vi "GetUser.vi"(10 "string":string caption="字符串", 11 "权限":string(combo)="QX01") -> (0 "员工姓名":string, 1 "权限":bool, 3 "员工ID":string)   [LabVIEW 2013]
uses:
  <vilib>/Utility/error.llb/whitespace.ctl
panel:
  in  "error in (no error)":errorcluster
  out "error out":errorcluster
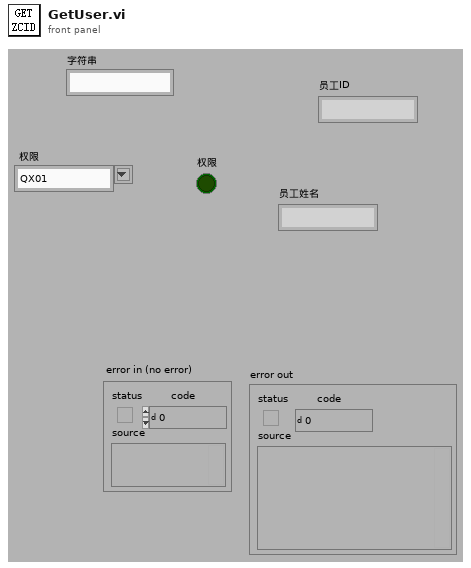
[diagram p1: front panel]
types:
  T1 = typedef "whitespace.ctl" = u16
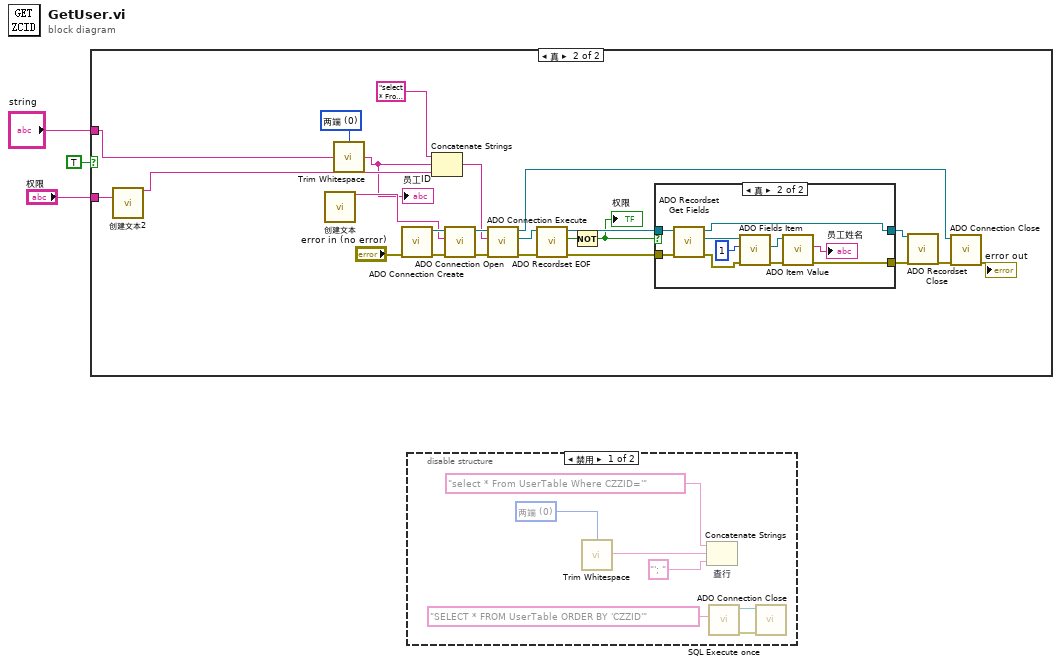
[diagram p0: block diagram]
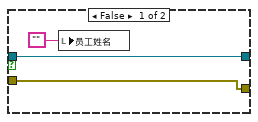
[diagram p3: hidden frame]
diagram:
  n1 = case shown="真" TRUE {
    tunnel: "权限" -> [_ w6]
    tunnel: "string" -> [_ w4]
    frame False {
    }
    frame True {
      w20 = T1 0 items=["两端", "字符串首端", "字符串末端"] ("location (both)")
      n2 = call "创建文本2"("权限"=w6) -> ("Result"=w7:string)  [unwired: 13 in, 1 out]
      n3 = call "创建文本"() -> ("Result"=w9:string)  [unwired: 14 in, 1 out]
      n4 = call <vilib>:"Trim Whitespace.vi"("string"=w4, "location (both)"=w20) -> ("trimmed string"=w5:string)
      "员工ID" <- w5
      n5 = call "ADO Connection Create.vi"("error in (no error)"="error in (no error)") -> ("error out"=w26:errorcluster, "ADODB._Connection Out"=w27:refnum<k7>)  [unwired: 9 out]
      n6 = Concatenate Strings ("查位置")("select * From UserTable Where  CZZID='" ("字符串 2"), w5, w7) -> (w10:string)
      n7 = call "ADO Connection Open.vi"("error in (no error)"=w26, "ConnectionString"=w9, "ADODB._Connection In"=w27) -> ("error out"=w25:errorcluster, "ADODB._Connection Out"=w11:refnum<k7>)  [unwired: 7 out]
      n8 = call "ADO Connection Execute.vi"("error in (no error)"=w25, "CommandText"=w10, "ADODB._Connection In"=w11) -> ("error out"=w23:errorcluster, "RecordSet"=w24:refnum<k7>, "ADODB._Connection Out"=w12:refnum<k7>)  [unwired: 6 out]
      n9 = call "ADO Recordset EOF.vi"("error in (no error)"=w23, "ADODB._Recordset In"=w24) -> ("error out"=w16:errorcluster, "EOF"=w13:bool, "ADODB._Recordset Out"=w17:refnum<k7>)  [unwired: 7 out]
      n10 = Not(x=w13) -> (.not. x?=w8:bool)
      "权限" <- w8
      n11 = case shown="真" w8 {
        tunnel: w17 -> [w29 w40]
        tunnel: w16 -> [w30 w39]
        tunnel: [w29 w38] -> w15
        tunnel: [w30 w32] -> w14
        frame False {
          n12 = local write "员工姓名"("") -> ()
        }
        frame True {
          n13 = call "ADO Recordset Get Fields.vi"("error in (no error)"=w39, "ADODB._Recordset In"=w40) -> ("error out"=w31:errorcluster, "Fields Out"=w37:refnum<k7>, "ADODB._Recordset Out"=w38:refnum<k7>)  [unwired: 7 out]
          n14 = call "ADO Fields Item.vi"("error in (no error)"=w31, "Index"=1, "Fields In"=w37) -> ("error out"=w35:errorcluster, "Item Out"=w34:refnum<k7>)  [unwired: 7 out]
          n15 = call "ADO Item Value.vi"("error in (no error)"=w35, "Item In"=w34) -> ("error out"=w32:errorcluster, "Value"=→"员工姓名":string)  [unwired: 8 out]
        }
      }
      n16 = call "ADO Recordset Close.vi"("ADODB._Recordset In"=w15, "error in (no error)"=w14) -> ("error out"=w22:errorcluster)  [unwired: 17 out]
      n17 = call "ADO Connection Close.vi"("error in (no error)"=w22, "ADODB._Connection In"=w12) -> ("error out"=→"error out":errorcluster)  [unwired: 9 out]
    }
  }
  n18 = disable-structure shown="禁用" {
    frame Disabled {
      w44 = T1 0 items=["两端", "字符串首端", "字符串末端"] ("location (both)")
      n19 = call <vilib>:"Trim Whitespace.vi"("location (both)"=w44) -> ("trimmed string"=w43:string)  [unwired: 1 in]
      n20 = Concatenate Strings "查行"("select * From UserTable Where CZZID='" ("字符串 2"), w43, "'; " ("字符串 2")) -> ()  [unwired: 1 out]
      n21 = call "SQL Execute once.vi"("Command Text"="SELECT * FROM UserTable ORDER BY 'CZZID'") -> ("error out"=w47:errorcluster, "ADODB._Connection Out"=w46:refnum<k7>)  [unwired: 3 in, 6 out]
      n22 = call "ADO Connection Close.vi"("error in (no error)"=w47, "ADODB._Connection In"=w46) -> ()  [unwired: 10 out]
    }
    frame Enabled {
    }
  }
